vi "Initiate Acquisition Core.vi"(8 "error in (no error)":errorcluster, 11 "CS++Scope":refnum<class "CS++Scope.lvclass">) -> (0 "error out":errorcluster, 3 "CS++Scope out":refnum<class "CS++Scope.lvclass">)   [LabVIEW 2013, in "CS++Scope.lvlib" / "CS++Scope.lvclass"]
doc: "This VI initiates a waveform acquisition. After you call this VI, the oscilloscope leaves the Idle state and waits for a trigger. The oscilloscope acquires a waveform for each channel you have enabled with the IviScope Configure Channel VI.\n\nNote (1) This VI does not check the instrument status. Typically, you call this VI only in a sequence of calls to other low-level driver VIs. The sequence performs one operation. You use the low-level VIs to optimize one or more aspects of interaction with the instrument. If you want to check the instrument status, call the IviScope Error-Query VI at the conclusion of the sequence.\n(2) This VI performs interchangeability checking when the IviScope>>Inherent IVI Settings>>User Options>>Interchange Check property is set to TRUE. If the IviScope>>Inherent IVI Settings>>User Options>>Spy property is set to TRUE, you use the NI I/O Trace utility to view interchangeability warnings. You use the IviScope Get Next Interchange Warning VI to retrieve interchangeability warnings when the IviScope>>Inherent IVI Settings>>User Options>>Spy property is set to FALSE. For more information about interchangeability checking, refer to the help text for the IviScope>>Inherent IVI Settings>>User Options>>Interchange Check property.\n(3) The class driver performs a simulated waveform acquisition when this VI is called and the IviScope>>Inherent IVI Settings>>User Options>>Simulate property is set to TRUE and the IviScope>>Inherent IVI Settings>>User Options>>Use Specific Simulation property is set to FALSE. For information on how to configure a simulated waveform, refer to the online help manual."
uses:
  CS++Scope.lvclass
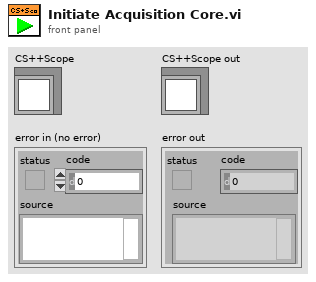
[diagram p1: front panel]
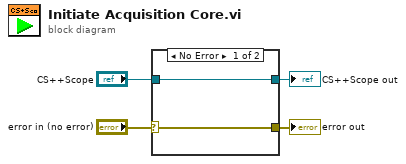
[diagram p0: block diagram]
diagram:
  n1 = case shown="No Error" "error in (no error)" {
    selector: "error in (no error)" -> [w5 w8]
    tunnel: [w5 w8] -> w3
    tunnel: [w6 w7] -> w2
    tunnel: "CS++Scope" -> [w6 w7]
    frame No Error {
    }
    frame Error {
    }
  }
  "error out" <- w3
  "CS++Scope out" <- w2
